vi "Lab Panel V6.00.vi"() -> ()   [LabVIEW 2017] (continued)
          n186 = local write "DISP LAB04-2"(w150) -> ()
        }
        frame #9 {
          w214 = 0
          w211 = FALSE
          # "initialise analog error control"
          n187 = local write "Resets Done"(0) -> ()
          n188 = local write "Auto Reset"(TRUE) -> ()
          n189 = local write "Er USB#0"(w214) -> ()
          n190 = local write "Er USB#1"(w214) -> ()
          n191 = local write "Er USB#2"(w214) -> ()
          n192 = local write "Analog error"(w211) -> ()
          n193 = local write "Reset Measuring"(w211) -> ()
          n194 = local write "Error USB #0"(w211) -> ()
          n195 = local write "Reset Error"(w211) -> ()
          n196 = local write "Error USB #1"(w211) -> ()
          n197 = local write "Error USB #2"(w211) -> ()
          n198 = local write "stop"(w211) -> ()
          n199 = local write "stop all"(w211) -> ()
        }
        frame #10 {
          # "get initial temperature values"
          n200 = stacked-sequence {
            frame #0 {
              w223 = T13 {"T1 Live"=20.0, "T1 Neut"=20.0, "T2 Live"=20.0, "T2 Neut"=20.0, "ID"=6.0, "ER"=10.0} ("LAB01 TEMP")
              n201 = local read "Select COM port"() -> (w218:refnum<visa-resource-name>)
              n202 = local write "LAB deg C"(w223) -> ()
              n203 = global write "Global display 4.vi" "LAB deg C"(w223) -> ()
              n204 = local write "OFF amps"(1.5) -> ()
              n205 = local write "ON amps"(20.0) -> ()
              n206 = local write "VOLTS"(250.0) -> ()
              n207 = local write "PF"(0.5) -> ()
              n208 = call "sub vi-open serial port v1.vi"("Select COM port"=w218) -> ("Error"=→"Com Port Status":bool, "LOOPS"=→"Com setup loops":i32, "VISA Com out"=→"VISA Com out":refnum<visa-resource-name>)  [unwired: 12 in]
            }
            frame #1 {
              n209 = for {
                N: 1 -> [_]
                w269 = TRUE
                n210 = local read "Temp Simulate"() -> (w225:bool)
                n211 = local write "Temp read loop"(0) -> ()
                n212 = case shown="True" w225 {
                  frame False {
                  }
                  frame True {
                    w271 = 20
                    n213 = local write "Ambient Volts"(2.92) -> ()
                    n214 = global write "Global display 3.vi" "Ref deg C"(w271) -> ()
                    n215 = local write "Ref deg C"(w271) -> ()
                  }
                }
                n216 = call "sub vi - GET ALL TEMP v7.vi"("LA01-EN"=w269, "LA02-EN"=w269, "LA03-EN"=w269, "LA04-EN"=w269, "LA05-EN"=w269, "simulate"=w225, "Gen Cal Value"=1) -> ("ID"=w231:T27, "LA01 TEMP"=w267:T28, "LA02 TEMP"=w260:T28, "LA04 TEMP"=w246:T28, "LA03 TEMP"=w253:T28, "LA05 TEMP"=w239:T28)  [unwired: 3 in, 4 out]
                n217 = local write "LAB05 TEMP"(w239) -> ()
                n218 = local write "LAB04 TEMP"(w246) -> ()
                n219 = Unbundle(w253) -> ("T1"=w250:dbl, "T2"=w249:dbl, "T3"=w248:dbl, "T4"=w247:dbl)  [unwired: 2 out]
                n220 = Unbundle(w267) -> ("T1"=w265:dbl, "T2"=w264:dbl, "T3"=w263:dbl, "T4"=w262:dbl)  [unwired: 2 out]
                n221 = Unbundle(w260) -> ("T1"=w257:dbl, "T2"=w256:dbl, "T3"=w255:dbl, "T4"=w254:dbl)  [unwired: 2 out]
                n222 = Unbundle(w246) -> ("T1"=w244:dbl, "T2"=w243:dbl, "T3"=w242:dbl, "T4"=w241:dbl)  [unwired: 2 out]
                n223 = Unbundle(w239) -> ("T1"=w237:dbl, "T2"=w236:dbl, "T3"=w235:dbl, "T4"=w234:dbl)  [unwired: 2 out]
                n224 = local write "LAB01 TEMP"(w267) -> ()
                n225 = local write "LAB02 TEMP"(w260) -> ()
                n226 = local write "LAB03 TEMP"(w253) -> ()
                n227 = Unbundle(w231) -> ("id1"=→"LAB01-TP":bool, "id2"=→"LAB02-TP":bool, "id3"=→"LAB03-TP":bool, "id4"=→"LAB04-TP":bool, "id5"=→"LAB05-TP":bool)
                n228 = local read "TEMP LA05"() -> (w238:T10)
                n229 = local read "TEMP LA04"() -> (w245:T10)
                n230 = local read "TEMP LA02"() -> (w259:T10)
                n231 = local read "TEMP LA03"() -> (w252:T10)
                n232 = local read "TEMP LA01"() -> (w266:T10)
                n233 = Bundle(cluster=w252, "TL-1"=w250, "TN-1"=w249, "TL-2"=w248, "TN-2"=w247) -> (w251:T10)  [unwired: 4 in]
                n234 = Bundle(cluster=w266, "TL-1"=w265, "TN-1"=w264, "TL-2"=w263, "TN-2"=w262) -> (w261:T10)  [unwired: 4 in]
                n235 = Bundle(cluster=w259, "TL-1"=w257, "TN-1"=w256, "TL-2"=w255, "TN-2"=w254) -> (w258:T10)  [unwired: 4 in]
                n236 = Bundle(cluster=w245, "TL-1"=w244, "TN-1"=w243, "TL-2"=w242, "TN-2"=w241) -> (w240:T10)  [unwired: 4 in]
                n237 = Bundle(cluster=w238, "TL-1"=w237, "TN-1"=w236, "TL-2"=w235, "TN-2"=w234) -> (w233:T10)  [unwired: 4 in]
                n238 = local write "TEMP LA03"(w251) -> ()
                n239 = local write "TEMP LA01"(w261) -> ()
                n240 = local write "TEMP LA02"(w258) -> ()
                n241 = local write "TEMP LA05"(w233) -> ()
                n242 = local write "TEMP LA04"(w240) -> ()
              }
            }
            frame #2 {
              w280 = 0
              n243 = local read "LAB01 TEMP"() -> (w282:T13)
              n244 = local read "SIG LAB01-2"() -> (w277:T2)
              n245 = Unbundle By Name(w282) -> ("T1 Live"=w275:dbl, "T1 Neut"=w274:dbl, "T2 Live"=w273:dbl, "T2 Neut"=w272:dbl)  [unwired: 2 out]
              n246 = local read "SIG LAB01-1"() -> (w279:T2)
              n247 = local read "TEMP LA01"() -> (w283:T10)
              n248 = Bundle By Name(cluster=w283, "TL-1"=w275, "TN-1"=w274, "TL-2"=w273, "TN-2"=w272, "TL -1COUNT"=w280, "TN-1 COUNT"=w280, "TL-2 COUNT"=w280, "TN-2 COUNT"=w280) -> (w281:T10)
              n249 = Bundle(cluster=w279, "Tmp Live"=w275, "Tmp Neut"=w274) -> (w278:T2)  [unwired: 3 in]
              n250 = Bundle(cluster=w277, "Tmp Live"=w273, "Tmp Neut"=w272) -> (w276:T2)  [unwired: 3 in]
              n251 = local write "SIG LAB01-2"(w276) -> ()
              n252 = local write "SIG LAB01-1"(w278) -> ()
              n253 = local write "TEMP LA01"(w281) -> ()
            }
            frame #3 {
              w292 = 0
              n254 = local read "LAB02 TEMP"() -> (w294:T13)
              n255 = Unbundle By Name(w294) -> ("T1 Live"=w287:dbl, "T1 Neut"=w286:dbl, "T2 Live"=w285:dbl, "T2 Neut"=w284:dbl)  [unwired: 2 out]
              n256 = local read "SIG LAB02-1"() -> (w291:T2)
              n257 = local read "SIG LAB02-2"() -> (w290:T2)
              n258 = local read "TEMP LA02"() -> (w295:T10)
              n259 = Bundle By Name(cluster=w295, "TL-1"=w287, "TN-1"=w286, "TL-2"=w285, "TN-2"=w284, "TL -1COUNT"=w292, "TN-1 COUNT"=w292, "TL-2 COUNT"=w292, "TN-2 COUNT"=w292) -> (w293:T10)
              n260 = Bundle(cluster=w290, "Tmp Live"=w285, "Tmp Neut"=w284) -> (w288:T2)  [unwired: 3 in]
              n261 = Bundle(cluster=w291, "Tmp Live"=w287, "Tmp Neut"=w286) -> (w289:T2)  [unwired: 3 in]
              n262 = local write "TEMP LA02"(w293) -> ()
              n263 = local write "SIG LAB02-1"(w289) -> ()
              n264 = local write "SIG LAB02-2"(w288) -> ()
            }
            frame #4 {
              w304 = 0
              n265 = local read "LAB03 TEMP"() -> (w306:T13)
              n266 = Unbundle By Name(w306) -> ("T1 Live"=w299:dbl, "T1 Neut"=w298:dbl, "T2 Live"=w297:dbl, "T2 Neut"=w296:dbl)  [unwired: 2 out]
              n267 = local read "SIG LAB03-1"() -> (w303:T2)
              n268 = local read "SIG LAB03-2"() -> (w302:T2)
              n269 = local read "TEMP LA03"() -> (w307:T10)
              n270 = Bundle By Name(cluster=w307, "TL-1"=w299, "TN-1"=w298, "TL-2"=w297, "TN-2"=w296, "TL -1COUNT"=w304, "TN-1 COUNT"=w304, "TL-2 COUNT"=w304, "TN-2 COUNT"=w304) -> (w305:T10)
              n271 = Bundle(cluster=w302, "Tmp Live"=w297, "Tmp Neut"=w296) -> (w300:T2)  [unwired: 3 in]
              n272 = Bundle(cluster=w303, "Tmp Live"=w299, "Tmp Neut"=w298) -> (w301:T2)  [unwired: 3 in]
              n273 = local write "TEMP LA03"(w305) -> ()
              n274 = local write "SIG LAB03-2"(w300) -> ()
              n275 = local write "SIG LAB03-1"(w301) -> ()
            }
            frame #5 {
              w316 = 0
              n276 = local read "LAB04 TEMP"() -> (w318:T13)
              n277 = Unbundle By Name(w318) -> ("T1 Live"=w311:dbl, "T1 Neut"=w310:dbl, "T2 Live"=w309:dbl, "T2 Neut"=w308:dbl)  [unwired: 2 out]
              n278 = local read "SIG LAB04-2"() -> (w314:T2)
              n279 = local read "SIG LAB04-1"() -> (w315:T2)
              n280 = local read "TEMP LA04"() -> (w319:T10)
              n281 = Bundle By Name(cluster=w319, "TL-1"=w311, "TN-1"=w310, "TL-2"=w309, "TN-2"=w308, "TL -1COUNT"=w316, "TN-1 COUNT"=w316, "TL-2 COUNT"=w316, "TN-2 COUNT"=w316) -> (w317:T10)
              n282 = Bundle(cluster=w314, "Tmp Live"=w309, "Tmp Neut"=w308) -> (w312:T2)  [unwired: 3 in]
              n283 = Bundle(cluster=w315, "Tmp Live"=w311, "Tmp Neut"=w310) -> (w313:T2)  [unwired: 3 in]
              n284 = local write "SIG LAB04-2"(w312) -> ()
              n285 = local write "TEMP LA04"(w317) -> ()
              n286 = local write "SIG LAB04-1"(w313) -> ()
            }
            frame #6 {
              w328 = 0
              n287 = local read "LAB05 TEMP"() -> (w330:T13)
              n288 = Unbundle By Name(w330) -> ("T1 Live"=w323:dbl, "T1 Neut"=w322:dbl, "T2 Live"=w321:dbl, "T2 Neut"=w320:dbl)  [unwired: 2 out]
              n289 = local read "SIG LAB05-2"() -> (w326:T2)
              n290 = local read "SIG LAB05-1"() -> (w327:T2)
              n291 = local read "TEMP LA05"() -> (w331:T10)
              n292 = Bundle By Name(cluster=w331, "TL-1"=w323, "TN-1"=w322, "TL-2"=w321, "TN-2"=w320, "TL -1COUNT"=w328, "TN-1 COUNT"=w328, "TL-2 COUNT"=w328, "TN-2 COUNT"=w328) -> (w329:T10)
              n293 = Bundle(cluster=w326, "Tmp Live"=w321, "Tmp Neut"=w320) -> (w324:T2)  [unwired: 3 in]
              n294 = Bundle(cluster=w327, "Tmp Live"=w323, "Tmp Neut"=w322) -> (w325:T2)  [unwired: 3 in]
              n295 = local write "SIG LAB05-2"(w324) -> ()
              n296 = local write "SIG LAB05-1"(w325) -> ()
              n297 = local write "TEMP LA05"(w329) -> ()
            }
          }
        }
        frame #11 {
          # "Create analog task"
          n298 = local read "DAQ Simulate"() -> (w333:bool)
          n299 = case shown="False" w333 {
            tunnel: w332 -> [w334 _]
            frame False {
              n300 = local read "RATE (Hz)"() -> (w341:dbl)
              n301 = local read "SAMPLES"() -> (w340:dbl)
              n302 = call "sub vi - AI USB4704 (3)  Create Task v4.vi"("Test"=w334, "Rate Hz"=w341, "Samples"=w340) -> ("physical channels 0"=→"physical channels 0":string, "physical channels 1"=→"physical channels 1":string, "physical channels 2"=→"physical channels 2":string, "TASK USB 0"=→"AI Task0":i32, "TASK USB 1"=→"AI Task1":i32, "TASK USB 2"=→"AI Task2":i32, "AI Task Er"=w338:bool)  [unwired: 5 in, 1 out]
              n303 = local write "Reset Error"(w338) -> ()
              "AI Task" <- TRUE
            }
            frame True {
            }
          }
        }
        frame #12 {
          # "Enable front panel, all settings done"
          n304 = property on="Tab Control 2" class="TabCtl (strict)"("DisabledEnum"=T17."Enabled" ("Disabled")) -> ()  [unwired: 2 in, 2 out]
          n305 = property on="Tab Control 2" class="TabCtl (strict)"("Value"=0) -> ()  [unwired: 2 in, 2 out]
        }
        frame #13 {
          n306 = property on="Tab Control 2" class="TabCtl (strict)"("Value"=0) -> ()  [unwired: 2 in, 2 out]
        }
      }
    }
    frame #2 {
      w349 = 250.0
      # "frames that only action on certain cycles, 13, 14, 15, 16, 19, 21"
      # "Main Loop"
      n307 = node-c288(w349) -> (w351:T19)  [unwired: 3 in]
      n308 = timed-loop {
        timing: w351 -> [_]
        timing-out: [_] -> w350
        tunnel: w349 -> [w353]
        tunnel: w348 -> [w352]
        i -> [w379]
        stop <- w354 stop-if-true
        n309 = node-c288() -> ()  [unwired: 1 in, 1 out]
        n310 = local read "Resets Done"() -> (w358:dbl)
        n311 = local read "SELECT LAB05-2"() -> (w359:T3)
        n312 = local read "SELECT LAB05-1"() -> (w360:T3)
        n313 = local read "SELECT LAB04-2"() -> (w361:T3)
        n314 = local read "SELECT LAB03-1"() -> (w364:T3)
        n315 = local read "SELECT LAB02-2"() -> (w365:T3)
        n316 = local read "SELECT LAB03-2"() -> (w363:T3)
        n317 = local read "SELECT LAB04-1"() -> (w362:T3)
        n318 = local read "SELECT LAB02-1"() -> (w366:T3)
        n319 = local read "run lab03-2"() -> (w373:bool)
        n320 = local read "run lab04-1"() -> (w372:bool)
        n321 = local read "run lab05-1"() -> (w370:bool)
        n322 = local read "run lab04-2"() -> (w371:bool)
        n323 = local read "run lab05-2"() -> (w369:bool)
        n324 = local read "run lab03-1"() -> (w374:bool)
        n325 = local read "run lab02-2"() -> (w375:bool)
        n326 = local read "SELECT LAB01-1"() -> (w368:T3)
        n327 = local read "SELECT LAB01-2"() -> (w367:T3)
        n328 = local read "run lab02-1"() -> (w376:bool)
        n329 = Greater?(x=w358, y=50) -> (0:w355:bool)
        n330 = Or(x=w355, y="stop") -> (x .or. y?=w354:bool)
        n331 = local read "run lab01-1"() -> (w378:bool)
        n332 = local read "run lab01-2"() -> (w377:bool)
        n333 = global write "Global display 1.vi" "stop disp"(w354) -> ()
        n334 = stacked-sequence {
          seq-local: [_ _ w496 _ _ _ _ _ _ _ _ _ _ _ _ _ _ _ _ _ _ _ _ _ _ _ _] -> [_ _ _ _ _ _ w2602 _ _ _ _ _ _ _ _ _ _ _ _ _ _ _ _ _ _ _ _]
          seq-local: [_ _ w495 _ _ _ _ _ _ _ _ _ _ _ _ _ _ _ _ _ _ _ _ _ _ _ _] -> [_ _ _ _ _ _ w2601 _ _ _ _ _ _ _ _ _ _ _ _ _ _ _ _ _ _ _ _]
          seq-local: [_ _ w482 _ _ _ _ _ _ _ _ _ _ _ _ _ _ _ _ _ _ _ _ _ _ _ _] -> [_ _ _ _ _ _ w2600 _ _ _ _ _ _ _ _ _ _ _ _ _ _ _ _ _ _ _ _]
          seq-local: [_ _ w481 _ _ _ _ _ _ _ _ _ _ _ _ _ _ _ _ _ _ _ _ _ _ _ _] -> [_ _ _ _ _ _ w2599 _ _ _ _ _ _ _ _ _ _ _ _ _ _ _ _ _ _ _ _]
          seq-local: [_ _ w480 _ _ _ _ _ _ _ _ _ _ _ _ _ _ _ _ _ _ _ _ _ _ _ _] -> [_ _ _ _ _ _ w2598 _ _ _ _ _ _ _ _ _ _ _ _ _ _ _ _ _ _ _ _]
          seq-local: [_ _ w479 _ _ _ _ _ _ _ _ _ _ _ _ _ _ _ _ _ _ _ _ _ _ _ _] -> [_ _ _ _ _ _ w2597 _ _ _ _ _ _ _ _ _ _ _ _ _ _ _ _ _ _ _ _]
          seq-local: [_ _ w478 _ _ _ _ _ _ _ _ _ _ _ _ _ _ _ _ _ _ _ _ _ _ _ _] -> [_ _ _ _ _ _ w2596 _ _ _ _ _ _ _ _ _ _ _ _ _ _ _ _ _ _ _ _]
          seq-local: [_ _ w477 _ _ _ _ _ _ _ _ _ _ _ _ _ _ _ _ _ _ _ _ _ _ _ _] -> [_ _ _ _ _ _ w2595 _ _ _ _ _ _ _ _ _ _ _ _ _ _ _ _ _ _ _ _]
          seq-local: [_ _ w476 _ _ _ _ _ _ _ _ _ _ _ _ _ _ _ _ _ _ _ _ _ _ _ _] -> [_ _ _ _ _ _ w2594 _ _ _ _ _ _ _ _ _ _ _ _ _ _ _ _ _ _ _ _]
          seq-local: [_ _ w475 _ _ _ _ _ _ _ _ _ _ _ _ _ _ _ _ _ _ _ _ _ _ _ _] -> [_ _ _ _ _ _ w2593 _ _ _ _ _ _ _ _ _ _ _ _ _ _ _ _ _ _ _ _]
          seq-local: [_ _ _ _ _ _ _ _ _ _ _ _ w3746 _ _ _ _ _ _ _ _ _ _ _ _ _ _] -> [_ _ _ _ _ _ _ _ _ _ _ _ _ w3783 _ _ _ _ _ _ _ _ _ _ _ _ _]
          seq-local: [w383 _ _ _ _ _ _ _ _ _ _ _ _ _ _ _ _ _ _ _ _ _ _ _ _ _ _] -> [_ _ _ _ _ _ _ _ _ _ _ _ _ _ _ _ _ _ _ _ _ _ _ _ _ _ w6492]
          tunnel: w378 -> [_ _ _ w513 w765 w2192 w2622 w2938 w3426 _ _ _ _ _ w4097 _ w5055 _ _ w5404 w5708 w5889 _ _ _ _ _]
          tunnel: w377 -> [_ _ _ w512 w763 w2191 w2621 w2939 w3425 _ _ _ _ _ w4096 _ w5053 _ _ w5403 w5707 w5887 _ _ _ _ _]
          tunnel: w376 -> [_ _ _ w511 w761 w2190 w2620 w2937 w3424 _ _ _ _ _ w4095 _ w5051 _ _ w5402 w5706 w5886 _ _ _ _ _]
          tunnel: w375 -> [_ _ _ w510 w759 w2189 w2619 w2936 w3423 _ _ _ _ _ w4094 _ w5049 _ _ w5401 w5705 w5885 _ _ _ _ _]
          tunnel: w374 -> [_ _ _ w509 w757 w2188 w2618 w2935 w3422 _ _ _ _ _ w4093 _ w5047 _ _ w5400 w5704 w5884 _ _ _ _ _]
          tunnel: w373 -> [_ _ _ w508 w755 w2187 w2617 w2934 w3421 _ _ _ _ _ w4092 _ w5045 _ _ w5399 w5703 w5883 _ _ _ _ _]
          tunnel: w372 -> [_ _ _ w507 w753 w2186 w2616 w2933 w3420 _ _ _ _ _ w4091 _ w5043 _ _ w5398 w5702 w5882 _ _ _ _ _]
          tunnel: w371 -> [_ _ _ w506 w751 w2185 w2615 w2932 w3419 _ _ _ _ _ w4090 _ w5041 _ _ w5397 w5701 w5881 _ _ _ _ _]
          tunnel: w370 -> [_ _ _ w505 w749 w2184 w2614 w2931 w3418 _ _ _ _ _ w4089 _ w5039 _ _ w5396 w5700 w5880 _ _ _ _ _]
          tunnel: w369 -> [_ _ _ w504 w747 w2183 w2613 w2930 w3417 _ _ _ _ _ w4088 _ w5037 _ _ w5395 w5699 w5879 _ _ _ _ _]
          tunnel: w368 -> [_ _ _ _ w764 w2182 w2612 _ _ _ _ _ _ _ _ _ w5057 _ _ _ _ _ w6352 _ _ _ _]
          tunnel: w367 -> [_ _ _ _ w762 w2181 w2611 _ _ _ _ _ _ _ _ _ w5052 _ _ _ _ _ w6351 _ _ _ _]
          tunnel: w366 -> [_ _ _ _ w760 w2180 w2610 _ _ _ _ _ _ _ _ _ w5050 _ _ _ _ _ w6350 _ _ _ _]
          tunnel: w365 -> [_ _ _ _ w758 w2179 w2609 _ _ _ _ _ _ _ _ _ w5048 _ _ _ _ _ w6349 _ _ _ _]
          tunnel: w364 -> [_ _ _ _ w756 w2178 w2608 _ _ _ _ _ _ _ _ _ w5046 _ _ _ _ _ w6348 _ _ _ _]
          tunnel: w363 -> [_ _ _ _ w754 w2177 w2607 _ _ _ _ _ _ _ _ _ w5044 _ _ _ _ _ w6347 _ _ _ _]
          tunnel: w362 -> [_ _ _ _ w752 w2176 w2606 _ _ _ _ _ _ _ _ _ w5042 _ _ _ _ _ w6346 _ _ _ _]
          tunnel: w361 -> [_ _ _ _ w750 w2175 w2605 _ _ _ _ _ _ _ _ _ w5040 _ _ _ _ _ w6345 _ _ _ _]
          tunnel: w360 -> [_ _ _ _ w748 w2174 w2604 _ _ _ _ _ _ _ _ _ w5038 _ _ _ _ _ w6344 _ _ _ _]
          tunnel: w359 -> [_ _ _ _ w746 w2173 w2603 _ _ _ _ _ _ _ _ _ w5036 _ _ _ _ _ w6343 _ _ _ _]
          tunnel: w355 -> [_ _ _ _ _ _ _ _ _ _ _ _ _ _ _ _ _ _ _ _ _ _ _ _ w6455 _ _]
          tunnel: w354 -> [_ _ _ _ _ _ _ _ _ _ _ _ _ _ _ _ _ _ _ _ _ _ _ _ w6454 _ _]
          tunnel: w353 -> [_ w428 _ _ _ _ _ _ _ _ _ _ _ _ _ _ _ _ _ _ _ _ _ _ _ _ _]
          tunnel: w352 -> [w382 _ _ w499 _ _ _ _ _ _ _ w3591 w3744 _ _ _ _ _ _ _ _ _ _ _ _ _ _]
          frame #0 {
            # "Acquire analog Inputs"
            n335 = Tick Count (ms)() -> (millisecond timer value=w383:u32)
            n336 = global write "Global 1.vi" "RATE(Hz)"("RATE (Hz)") -> ()
            n337 = local read "AI Task"() -> (w385:bool)
            n338 = case shown="True" w385 {
              tunnel: "RATE (Hz)" -> [_ _]
              tunnel: w382 -> [_ w394]
              tunnel: w382 -> [_ w393]
              frame False {
              }
              frame True {
                n339 = Tick Count (ms)() -> (millisecond timer value=w398:u32)
                n340 = flat-sequence {
                  tunnel: w398 -> [w400]
                  tunnel: [w400] -> w397
                  tunnel: w394 -> [w399]
                  tunnel: w397 -> [w409]
                  tunnel: [w407] -> w395
                  tunnel: [w414] -> w396
                  tunnel: w395 -> [w414]
                  tunnel: w393 -> [w412]
                  tunnel: w396 -> [w425]
                  frame #0 {
                    n341 = disable-structure shown="Disabled" {
                      disable-tunnel: w399 -> [w401 _]
                      frame Disabled {
                        n342 = local read "RATE (Hz)"() -> (w406:dbl)
                        n343 = local read "SAMPLES"() -> (w405:dbl)
                        n344 = call "sub vi - AI USB4704 (3)  Create Task v4.vi"("Test"=w401, "Rate Hz"=w406, "Samples"=w405) -> ("TASK USB 0"=w403:i32, "TASK USB 1"=w404:i32, "TASK USB 2"=w402:i32)  [unwired: 5 in, 5 out]
                        n345 = local write "AI Task0"(w403) -> ()
                        n346 = local write "AI Task1"(w404) -> ()
                        n347 = local write "AI Task2"(w402) -> ()
                      }
                      frame Enabled {
                      }
                    }
                  }
                  frame #1 {
                    n348 = Tick Count (ms)() -> (millisecond timer value=w407:u32)
                    n349 = Subtract(x=w407, y=w409) -> (x-y=→"ACQ Init TIme":u32)
                  }
                  frame #2 {
                    n350 = local read "SAMPLES"() -> (w415:dbl)
                    n351 = local read "AI Task0"() -> (w423:u64)
                    n352 = local read "AI Task1"() -> (w422:u32)
                    n353 = local read "AI Task2"() -> (w421:u32)
                    n354 = local read "MAIL SETTINGS"() -> (w413:T8)
                    n355 = call "sub vi - AI USB4704 (3) v73.vi"("Task0"=w423, "Test"=w412, "Task1"=w422, "Task2"=w421, "SAMPLES"=w415, "MAIL SETTINGS"=w413) -> ("Fault"=w410:bool, "data 0"=→"AI data 0" →"AI Data 0":waveform(dbl)[], "data 1"=→"AI data 1" →"AI Data 1":waveform(dbl)[], "data 2"=→"AI data 2" →"AI Data 2":waveform(dbl)[], "loop time"=→"AI loop time":dbl, "Fault Counts"=→"Analog Fault Counts":i32[], "error array"=→"AI Error":errorcluster[])  [unwired: 3 in]
                    n356 = local write "Analog error"(w410) -> ()
                  }
                  frame #3 {
                    n357 = Tick Count (ms)() -> (millisecond timer value=w426:u32)
                    n358 = Tick Count (ms)() -> ()  [unwired: 1 out]
                    n359 = Subtract(x=w426, y=w425) -> (x-y=→"ACQ Time":u32)
                  }
                }
              }
            }
            n360 = disable-structure shown="Disabled" {
              frame Disabled {
                n361 = call <userlib>:"Periodic Trigger__ogtk.vi"("time (ms)"=u32 1000) -> ("Triggered"=w387:bool)  [unwired: 12 in, 2 out]
                n362 = case shown="True" w387 {
                  frame False {
                  }
                  frame True {
                    n363 = control-ref of="This VI"() -> (w392:refnum<vi>)
                    n364 = invoke class="VI" method="FP.Get Image"(reference=w392) -> ("image data"=w391:T29)  [unwired: 5 in, 5 out]
                    n365 = Build Path(base path="path to JPEG file", name or relative path="FP.jpg") -> (appended path=w388:path)
                    n366 = call <vilib>:"Write JPEG File.vi"("image data"=w391, "path to JPEG file"=w388) -> ()  [unwired: 8 in, 2 out]
                  }
                }
              }
              frame Enabled {
              }
            }
          }
          frame #1 {
            w435 = FALSE
            # "Loop time (s)"
            # "set up cycle control"
            n367 = local read "jig cycle"() -> (w439:dbl)
            n368 = local read "Amps Fail level"() -> (w433:dbl)
            n369 = Divide(x=w428, y=1000.0) -> (x/y=w427:dbl)
            n370 = local read "DAQ Simulate"() -> (w430:bool)
            n371 = Divide(x="JIG ON TIME (S)", y=w427) -> (x/y=→"on loops":dbl)
            n372 = Divide(x="JIG OFF TIME (S)", y=w427) -> (x/y=→"off loops":dbl)
            n373 = Increment(x=w439) -> (x+1=w438:dbl)
            n374 = local write "Simulate IND"(w430) -> ()
            n375 = global write "Global display 3.vi" "Amps Fail"(w433) -> ()
            n376 = local write "TEMP"(w435) -> ()
            n377 = local write "AI"(w435) -> ()
            n378 = local read "Network Directory"() -> (w432:path)
            n379 = local write "jig cycle"(w438) -> ()
            n380 = call "sub vi - check network dir v2.vi"("PATH"=w432) -> ("error"=w431:bool)  [unwired: 10 in]
            n381 = disable-structure shown="Enabled" {
              frame Enabled {
                n382 = property on="Tab Control 2" class="TabCtl (strict)"() -> ("Pages"=w443:refnum<vi>[])  [unwired: 2 in, 2 out]
                n383 = Index Array(array=w443, index=8) -> (element=w445:refnum<vi>)
                n384 = property class="Page"(reference=w445, "PageVis"=TRUE) -> ()  [unwired: 1 in, 2 out]
              }
              frame Disabled {
              }
            }
            n385 = global write "Global display 3.vi" "network drive"(w431) -> ()
            n386 = event shown="[1] \"ADMIN\": Value Change" {
              selector: _ -> [_ _]
              dyn-events: _ -> [_ _]
              timeout: 10 -> [_ _]
              event Timeout {
                n387 = event-data() -> ()  [unwired: 1 in, 3 out]
              }
              event "ADMIN": Value Change {
                n388 = event-data() -> ()  [unwired: 1 in, 6 out]
                n389 = stacked-sequence {
                  seq-local: [_ w447 _] -> [_ _ w448]
                  frame #0 {
                    n390 = global write "Global 1.vi" "password"("9949") -> ()
                  }
                  frame #1 {
                    n391 = call "sub vi - password 1.vi"() -> ("RESULT"=w447:bool)  [unwired: 11 in]
                  }
                  frame #2 {
                    w450 = FALSE
                    n392 = property on="Tab Control 2" class="TabCtl (strict)"() -> ("Pages"=w454:refnum<vi>[])  [unwired: 2 in, 2 out]
                    n393 = Select(t=TRUE, s=w448, f=w450) -> (s? t:f=w449:bool)
                    n394 = Index Array(array=w454, index=8) -> (element=w452:refnum<vi>)
                    n395 = property class="Page"(reference=w452, "PageVis"=w449) -> ()  [unwired: 1 in, 2 out]
                    n396 = local write "ADMIN"(w450) -> ()
                  }
                }
              }
            }
            n397 = local write "network error"(w431) -> ()
          }
          frame #2 {
            w492 = 60.0
            # "Test Cycles"
            # "seconds"
            # "convert temperature rise minutes to cycles"
            n398 = local read "SET LAB05-2"() -> (w456:T5)
            n399 = local read "SET LAB05-1"() -> (w458:T5)
            n400 = local read "SET LAB04-2"() -> (w460:T5)
            n401 = local read "SET LAB01-1"() -> (w474:T6)
            n402 = local read "SET LAB01-2"() -> (w472:T5)
            n403 = local read "SET LAB02-2"() -> (w468:T5)
            n404 = local read "SET LAB04-1"() -> (w462:T5)
            n405 = local read "SET LAB03-1"() -> (w466:T5)
            n406 = local read "SET LAB03-2"() -> (w464:T5)
            n407 = local read "SET LAB02-1"() -> (w470:T5)
            n408 = local read "JIG OFF TIME (S)"() -> (w497:dbl)
            n409 = local read "JIG ON TIME (S)"() -> (w498:dbl)
            n410 = Unbundle By Name(w474) -> ("T-RISE mins"=w473:dbl)
            n411 = Unbundle(w456) -> ("T-RISE mins"=w455:dbl)  [unwired: 4 out]
            n412 = Unbundle(w458) -> ("T-RISE mins"=w457:dbl)  [unwired: 4 out]
            n413 = Unbundle(w460) -> ("T-RISE mins"=w459:dbl)  [unwired: 4 out]
            n414 = Unbundle(w472) -> ("T-RISE mins"=w471:dbl)  [unwired: 4 out]
            n415 = Unbundle(w470) -> ("T-RISE mins"=w469:dbl)  [unwired: 4 out]
            n416 = Unbundle(w462) -> ("T-RISE mins"=w461:dbl)  [unwired: 4 out]
            n417 = Unbundle(w468) -> ("T-RISE mins"=w467:dbl)  [unwired: 4 out]
            n418 = Unbundle(w464) -> ("T-RISE mins"=w463:dbl)  [unwired: 4 out]
            n419 = Unbundle(w466) -> ("T-RISE mins"=w465:dbl)  [unwired: 4 out]
            n420 = Add(x=w498, y=w497) -> (x+y=w491:dbl)
            n421 = Multiply(x=w492, y=w463) -> (x*y=w487:dbl)
            n422 = Multiply(x=w492, y=w461) -> (x*y=w486:dbl)
            n423 = Multiply(x=w492, y=w459) -> (x*y=w485:dbl)
            n424 = Multiply(x=w492, y=w457) -> (x*y=w484:dbl)
            n425 = Multiply(x=w492, y=w455) -> (x*y=w483:dbl)
            n426 = Multiply(x=w492, y=w471) -> (x*y=w493:dbl)
            n427 = Multiply(x=w492, y=w465) -> (x*y=w488:dbl)
            n428 = Multiply(x=w492, y=w473) -> (x*y=w494:dbl)
            n429 = Multiply(x=w492, y=w469) -> (x*y=w490:dbl)
            n430 = Multiply(x=w492, y=w467) -> (x*y=w489:dbl)
            n431 = Divide(x=w484, y=w491) -> (x/y=w476:dbl)
            n432 = Divide(x=w485, y=w491) -> (x/y=w477:dbl)
            n433 = Divide(x=w486, y=w491) -> (x/y=w478:dbl)
            n434 = Divide(x=w483, y=w491) -> (x/y=w475:dbl)
            n435 = Divide(x=w488, y=w491) -> (x/y=w480:dbl)
            n436 = Divide(x=w494, y=w491) -> (x/y=w496:dbl)
            n437 = Divide(x=w493, y=w491) -> (x/y=w495:dbl)
            n438 = Divide(x=w490, y=w491) -> (x/y=w482:dbl)
            n439 = Divide(x=w489, y=w491) -> (x/y=w481:dbl)
            n440 = Divide(x=w487, y=w491) -> (x/y=w479:dbl)
          }
          frame #3 {
            # "control cycle loops"
            n441 = local read "JIG OFF TIME (S)"() -> (w502:dbl)
            n442 = local read "JIG ON TIME (S)"() -> (w501:dbl)
            n443 = local read "on loops"() -> (w517:dbl)
            n444 = local read "off loops"() -> (w516:dbl)
            n445 = local read "jig cycle"() -> (w515:dbl)
            n446 = Add(x=w502, y=w501) -> (x+y=w500:dbl)
            n447 = Add(x=w517, y=w516) -> (x+y=w503:dbl)
            n448 = Greater Or Equal?(x=w515, y=w503) -> (x >= y?=w514:bool)
            n449 = case shown="True" w514 {
              tunnel: w513 -> [_ w552]
              tunnel: w512 -> [_ w551]
              tunnel: w511 -> [_ w550]
              tunnel: w510 -> [_ w549]
              tunnel: w509 -> [_ w548]
              tunnel: w508 -> [_ w547]
              tunnel: w507 -> [_ w546]
              tunnel: w506 -> [_ w545]
              tunnel: w505 -> [_ w544]
              tunnel: w504 -> [_ w543]
              tunnel: w500 -> [_ w542]
              tunnel: w499 -> [_ w518]
              frame False {
              }
              frame True {
                # "increment cycle value and convert cycles to minutes for temp rise"
                n450 = stacked-sequence {
                  tunnel: w518 -> [_ w556]
                  frame #0 {
                    n451 = local read "Temp read loop"() -> (w555:dbl)
                    n452 = Increment(x=w555) -> (x+1=w554:dbl)
                    n453 = local write "Temp read loop"(w554) -> ()
                  }
                  frame #1 {
                    n454 = case shown="True" w556 {
                      tunnel: [20 2] -> w558
                      frame False {
                      }
                      frame True {
                      }
                    }
                    n455 = local read "Temp read loop"() -> (w557:dbl)
                    n456 = Greater?(x=w557, y=w558) -> (0:w559:bool)
                    n457 = case shown="True" w559 {
                      frame False {
                      }
                      frame True {
                        n458 = local write "Temp read loop"(1) -> ()
                      }
                    }
                  }
                }
                n459 = local read "JIG RELAY CYCLES"() -> (w541:T9)
                n460 = local read "Temp read loop"() -> (→"Temp Up":dbl)
                n461 = Unbundle By Name(w541) -> ("LAB01-1"=w539:dbl, "LAB01-2"=w537:dbl, "LAB02-1"=w535:dbl, "LAB02-2"=w533:dbl, "LAB03-1"=w531:dbl, "LAB03-2"=w529:dbl, "LAB04-1"=w527:dbl, "LAB04-2"=w525:dbl, "LAB05-1"=w523:dbl, "LAB05-2"=w521:dbl)
                n462 = stacked-sequence {
                  tunnel: w552 -> [w573 _ _ _ _ _ _ _ _ _]
                  tunnel: w551 -> [_ w590 _ _ _ _ _ _ _ _]
                  tunnel: w550 -> [_ _ w607 _ _ _ _ _ _ _]
                  tunnel: w549 -> [_ _ _ w624 _ _ _ _ _ _]
                  tunnel: w548 -> [_ _ _ _ w641 _ _ _ _ _]
                  tunnel: w547 -> [_ _ _ _ _ w658 _ _ _ _]
                  tunnel: w546 -> [_ _ _ _ _ _ w675 _ _ _]
                  tunnel: w545 -> [_ _ _ _ _ _ _ w692 _ _]
                  tunnel: w544 -> [_ _ _ _ _ _ _ _ w709 _]
                  tunnel: w543 -> [_ _ _ _ _ _ _ _ _ w726]
                  tunnel: w542 -> [w570 w587 w604 w621 w638 w655 w672 w689 w706 w723]
                  tunnel: w539 -> [w564 _ _ _ _ _ _ _ _ _]
                  tunnel: [w563 _ _ _ _ _ _ _ _ _] -> w538
                  tunnel: w537 -> [_ w581 _ _ _ _ _ _ _ _]
                  tunnel: [_ w580 _ _ _ _ _ _ _ _] -> w536
                  tunnel: w535 -> [_ _ w598 _ _ _ _ _ _ _]
                  tunnel: [_ _ w597 _ _ _ _ _ _ _] -> w534
                  tunnel: w533 -> [_ _ _ w615 _ _ _ _ _ _]
                  tunnel: [_ _ _ w614 _ _ _ _ _ _] -> w532
                  tunnel: w531 -> [_ _ _ _ w632 _ _ _ _ _]
                  tunnel: [_ _ _ _ w631 _ _ _ _ _] -> w530
                  tunnel: w529 -> [_ _ _ _ _ w649 _ _ _ _]
                  tunnel: [_ _ _ _ _ w648 _ _ _ _] -> w528
                  tunnel: w527 -> [_ _ _ _ _ _ w666 _ _ _]
                  tunnel: [_ _ _ _ _ _ w665 _ _ _] -> w526
                  tunnel: w525 -> [_ _ _ _ _ _ _ w683 _ _]
                  tunnel: [_ _ _ _ _ _ _ w682 _ _] -> w524
                  tunnel: w523 -> [_ _ _ _ _ _ _ _ w700 _]
                  tunnel: [_ _ _ _ _ _ _ _ w699 _] -> w522
                  tunnel: w521 -> [_ _ _ _ _ _ _ _ _ w717]
                  tunnel: [_ _ _ _ _ _ _ _ _ w716] -> w520
                  frame #0 {
                    n463 = local read "DISP LAB01-1"() -> (w568:T4)
                    n464 = Unbundle By Name(w568) -> ("CYCLE"=w569:dbl)
                    n465 = case shown="True" w573 {
                      tunnel: w569 -> [w575 w579]
                      tunnel: [w575 w578] -> w567
                      tunnel: w564 -> [w574 w577]
                      tunnel: [w574 w576] -> w563
                      frame False {
                      }
                      frame True {
                        n466 = Increment(x=w577) -> (x+1=w576:dbl)
                        n467 = Increment(x=w579) -> (x+1=w578:dbl)
                      }
                    }
                    n468 = Multiply(x=w567, y=w570) -> (x*y=w571:dbl)
                    n469 = Divide(x=w571, y=60.0) -> (x/y=w566:dbl)
                    n470 = Bundle By Name(cluster=w568, "CYCLE"=w567, "MINS"=w566) -> (w565:T4)
                    n471 = local write "DISP LAB01-1"(w565) -> ()
                  }
                  frame #1 {
                    n472 = local read "DISP LAB01-2"() -> (w585:T4)
                    n473 = Unbundle By Name(w585) -> ("CYCLE"=w586:dbl)
                    n474 = case shown="True" w590 {
                      tunnel: w586 -> [w592 w596]
                      tunnel: [w592 w595] -> w583
                      tunnel: w581 -> [w591 w594]
                      tunnel: [w591 w593] -> w580
                      frame False {
                      }
                      frame True {
                        n475 = Increment(x=w594) -> (x+1=w593:dbl)
                        n476 = Increment(x=w596) -> (x+1=w595:dbl)
                      }
                    }
                    n477 = Multiply(x=w583, y=w587) -> (x*y=w588:dbl)
                    n478 = Divide(x=w588, y=60.0) -> (x/y=w582:dbl)
                    n479 = Bundle By Name(cluster=w585, "CYCLE"=w583, "MINS"=w582) -> (w584:T4)
                    n480 = local write "DISP LAB01-2"(w584) -> ()
                  }
                  frame #2 {
                    n481 = local read "DISP LAB02-1"() -> (w602:T4)
                    n482 = Unbundle By Name(w602) -> ("CYCLE"=w603:dbl)
                    n483 = case shown="True" w607 {
                      tunnel: [w609 w613] -> w600
                      tunnel: w603 -> [w609 w612]
                      tunnel: w598 -> [w608 w611]
                      tunnel: [w608 w610] -> w597
                      frame False {
                      }
                      frame True {
                        n484 = Increment(x=w611) -> (x+1=w610:dbl)
                        n485 = Increment(x=w612) -> (x+1=w613:dbl)
                      }
                    }
                    n486 = Multiply(x=w600, y=w604) -> (x*y=w605:dbl)
                    n487 = Divide(x=w605, y=60.0) -> (x/y=w599:dbl)
                    n488 = Bundle By Name(cluster=w602, "CYCLE"=w600, "MINS"=w599) -> (w601:T4)
                    n489 = local write "DISP LAB02-1"(w601) -> ()
                  }
                  frame #3 {
                    n490 = local read "DISP LAB02-2"() -> (w619:T4)
                    n491 = Unbundle By Name(w619) -> ("CYCLE"=w620:dbl)
                    n492 = case shown="True" w624 {
                      tunnel: [w626 w630] -> w618
                      tunnel: w620 -> [w626 w629]
                      tunnel: w615 -> [w625 w628]
                      tunnel: [w625 w627] -> w614
                      frame False {
                      }
                      frame True {
                        n493 = Increment(x=w628) -> (x+1=w627:dbl)
                        n494 = Increment(x=w629) -> (x+1=w630:dbl)
                      }
                    }
                    n495 = Multiply(x=w618, y=w621) -> (x*y=w622:dbl)
                    n496 = Divide(x=w622, y=60.0) -> (x/y=w617:dbl)
                    n497 = Bundle By Name(cluster=w619, "CYCLE"=w618, "MINS"=w617) -> (w616:T4)
                    n498 = local write "DISP LAB02-2"(w616) -> ()
                  }
                  frame #4 {
                    n499 = local read "DISP LAB03-1"() -> (w636:T4)
                    n500 = Unbundle(w636) -> ("CYCLE"=w637:dbl)  [unwired: 2 out]
                    n501 = case shown="True" w641 {
                      tunnel: [w643 w647] -> w633
                      tunnel: w637 -> [w643 w646]
                      tunnel: w632 -> [w642 w645]
                      tunnel: [w642 w644] -> w631
                      frame False {
                      }
                      frame True {
                        n502 = Increment(x=w645) -> (x+1=w644:dbl)
                        n503 = Increment(x=w646) -> (x+1=w647:dbl)
                      }
                    }
                    n504 = Multiply(x=w633, y=w638) -> (x*y=w639:dbl)
                    n505 = Divide(x=w639, y=60.0) -> (x/y=w634:dbl)
                    n506 = Bundle(cluster=w636, "CYCLE"=w633, "MINS"=w634) -> (w635:T4)  [unwired: 1 in]
                    n507 = local write "DISP LAB03-1"(w635) -> ()
                  }
                  frame #5 {
                    n508 = local read "DISP LAB03-2"() -> (w653:T4)
                    n509 = Unbundle(w653) -> ("CYCLE"=w654:dbl)  [unwired: 2 out]
                    n510 = case shown="True" w658 {
                      tunnel: [w660 w664] -> w652
                      tunnel: w654 -> [w660 w663]
                      tunnel: w649 -> [w659 w662]
                      tunnel: [w659 w661] -> w648
                      frame False {
                      }
                      frame True {
                        n511 = Increment(x=w662) -> (x+1=w661:dbl)
                        n512 = Increment(x=w663) -> (x+1=w664:dbl)
                      }
                    }
                    n513 = Multiply(x=w652, y=w655) -> (x*y=w656:dbl)
                    n514 = Divide(x=w656, y=60.0) -> (x/y=w651:dbl)
                    n515 = Bundle(cluster=w653, "CYCLE"=w652, "MINS"=w651) -> (w650:T4)  [unwired: 1 in]
                    n516 = local write "DISP LAB03-2"(w650) -> ()
                  }
                  frame #6 {
                    n517 = local read "DISP LAB04-1"() -> (w670:T4)
                    n518 = Unbundle(w670) -> ("CYCLE"=w671:dbl)  [unwired: 2 out]
                    n519 = case shown="True" w675 {
                      tunnel: [w677 w681] -> w668
                      tunnel: w671 -> [w677 w680]
                      tunnel: w666 -> [w676 w679]
                      tunnel: [w676 w678] -> w665
                      frame False {
                      }
                      frame True {
                        n520 = Increment(x=w679) -> (x+1=w678:dbl)
                        n521 = Increment(x=w680) -> (x+1=w681:dbl)
                      }
                    }
                    n522 = Multiply(x=w668, y=w672) -> (x*y=w673:dbl)
                    n523 = Divide(x=w673, y=60.0) -> (x/y=w667:dbl)
                    n524 = Bundle(cluster=w670, "CYCLE"=w668, "MINS"=w667) -> (w669:T4)  [unwired: 1 in]
                    n525 = local write "DISP LAB04-1"(w669) -> ()
                  }
                  frame #7 {
                    n526 = local read "DISP LAB04-2"() -> (w687:T4)
                    n527 = Unbundle(w687) -> ("CYCLE"=w688:dbl)  [unwired: 2 out]
                    n528 = case shown="True" w692 {
                      tunnel: [w694 w698] -> w685
                      tunnel: w688 -> [w694 w697]
                      tunnel: w683 -> [w693 w696]
                      tunnel: [w693 w695] -> w682
                      frame False {
                      }
                      frame True {
                        n529 = Increment(x=w696) -> (x+1=w695:dbl)
                        n530 = Increment(x=w697) -> (x+1=w698:dbl)
                      }
                    }
                    n531 = Multiply(x=w685, y=w689) -> (x*y=w691:dbl)
                    n532 = Divide(x=w691, y=60.0) -> (x/y=w684:dbl)
                    n533 = Bundle(cluster=w687, "CYCLE"=w685, "MINS"=w684) -> (w686:T4)  [unwired: 1 in]
                    n534 = local write "DISP LAB04-2"(w686) -> ()
                  }
                  frame #8 {
                    n535 = local read "DISP LAB05-1"() -> (w704:T4)
                    n536 = Unbundle(w704) -> ("CYCLE"=w705:dbl)  [unwired: 2 out]
                    n537 = case shown="True" w709 {
                      tunnel: [w711 w715] -> w702
                      tunnel: w705 -> [w711 w714]
                      tunnel: w700 -> [w710 w713]
                      tunnel: [w710 w712] -> w699
                      frame False {
                      }
                      frame True {
                        n538 = Increment(x=w713) -> (x+1=w712:dbl)
                        n539 = Increment(x=w714) -> (x+1=w715:dbl)
                      }
                    }
                    n540 = Multiply(x=w702, y=w706) -> (x*y=w707:dbl)
                    n541 = Divide(x=w707, y=60.0) -> (x/y=w701:dbl)
                    n542 = Bundle(cluster=w704, "CYCLE"=w702, "MINS"=w701) -> (w703:T4)  [unwired: 1 in]
                    n543 = local write "DISP LAB05-1"(w703) -> ()
                  }
                  frame #9 {
                    n544 = local read "DISP LAB05-2"() -> (w722:T4)
                    n545 = Unbundle(w722) -> ("CYCLE"=w721:dbl)  [unwired: 2 out]
                    n546 = case shown="True" w726 {
                      tunnel: [w728 w732] -> w720
                      tunnel: w721 -> [w728 w731]
                      tunnel: w717 -> [w727 w730]
                      tunnel: [w727 w729] -> w716
                      frame False {
                      }
                      frame True {
                        n547 = Increment(x=w730) -> (x+1=w729:dbl)
                        n548 = Increment(x=w731) -> (x+1=w732:dbl)
                      }
                    }
                    n549 = Multiply(x=w720, y=w723) -> (x*y=w724:dbl)
                    n550 = Divide(x=w724, y=60.0) -> (x/y=w719:dbl)
                    n551 = Bundle(cluster=w722, "CYCLE"=w720, "MINS"=w719) -> (w718:T4)  [unwired: 1 in]
                    n552 = local write "DISP LAB05-2"(w718) -> ()
                  }
                }
                n553 = local write "jig cycle"(0) -> ()
                n554 = Bundle By Name(cluster=w541, "LAB01-1"=w538, "LAB01-2"=w536, "LAB02-1"=w534, "LAB02-2"=w532, "LAB03-1"=w530, "LAB03-2"=w528, "LAB04-1"=w526, "LAB04-2"=w524, "LAB05-1"=w522, "LAB05-2"=w520) -> (w540:T9)
                n555 = local write "JIG RELAY CYCLES"(w540) -> ()
              }
            }
          }
          frame #4 {
            # "Note : Run lab0X-N variables are set which are written to digital I/O in frame 11"
            # "Why are these here?"
            # "START & STOP test RUN switch change, start test if true and stop test if false"
            n556 = Get Date/Time In Seconds() -> (seconds since 1Jan1904=w744:timestamp)
            n557 = local read "C drive data root dir"() -> (w737:path)
            n558 = Format Date/Time String(time format string (%c)="%b\\%a%d", seconds (now)=w744) -> (date/time string=w768:string)  [unwired: 1 in]
            n559 = Format Date/Time String(time format string (%c)="%H%M", seconds (now)=w744) -> (date/time string=w766:string)  [unwired: 1 in]
            n560 = Format Date/Time String(time format string (%c)="LabPanel%Y", seconds (now)=w744) -> (date/time string=w743:string)  [unwired: 1 in]
            n561 = Path To String(path=w737) -> (string=w740:string)
            n562 = global write "Global 1.vi" "C drive root path"(w737) -> ()
            n563 = local read "Ref deg C"() -> (w733:dbl)
            n564 = Concatenate Strings(w740, "\\") -> (w738:string)
            n565 = event shown="[1] \"RUN LAB01-1\": Value Change" {
              selector: _ -> [_ _ _ _ _ _ _ _ _ _ _]
              dyn-events: _ -> [_ _ _ _ _ _ _ _ _ _ _]
              timeout: 10 -> [_ _ _ _ _ _ _ _ _ _ _]
              tunnel: w738 -> [_ w781 w921 w1062 w1202 w1342 w1482 w1622 w1762 w1902 w2043]
              tunnel: w768 -> [_ w780 w920 w1061 w1201 w1341 w1481 w1621 w1761 w1901 w2042]
              tunnel: w766 -> [_ w778 w919 w1060 w1200 w1340 w1480 w1620 w1760 w1900 w2041]
              tunnel: w764 -> [_ w779 _ _ _ _ _ _ _ _ _]
              tunnel: w765 -> [_ _ _ _ _ _ _ _ _ _ _]
              tunnel: w763 -> [_ _ _ _ _ _ _ _ _ _ _]
              tunnel: w762 -> [_ _ w918 _ _ _ _ _ _ _ _]
              tunnel: w761 -> [_ _ _ _ _ _ _ _ _ _ _]
              tunnel: w760 -> [_ _ _ w1059 _ _ _ _ _ _ _]
              tunnel: w759 -> [_ _ _ _ _ _ _ _ _ _ _]
              tunnel: w758 -> [_ _ _ _ w1199 _ _ _ _ _ _]
              tunnel: w757 -> [_ _ _ _ _ _ _ _ _ _ _]
              tunnel: w756 -> [_ _ _ _ _ w1339 _ _ _ _ _]
              tunnel: w755 -> [_ _ _ _ _ _ _ _ _ _ _]
              tunnel: w754 -> [_ _ _ _ _ _ w1479 _ _ _ _]
              tunnel: w753 -> [_ _ _ _ _ _ _ _ _ _ _]
              tunnel: w752 -> [_ _ _ _ _ _ _ w1619 _ _ _]
              tunnel: w751 -> [_ _ _ _ _ _ _ _ _ _ _]
              tunnel: w750 -> [_ _ _ _ _ _ _ _ w1759 _ _]
              tunnel: w749 -> [_ _ _ _ _ _ _ _ _ _ _]
              tunnel: w748 -> [_ _ _ _ _ _ _ _ _ w1899 _]
              tunnel: w747 -> [_ _ _ _ _ _ _ _ _ _ _]
              tunnel: w746 -> [_ _ _ _ _ _ _ _ _ _ w2040]
              tunnel: w743 -> [_ w777 w917 w1058 w1198 w1338 w1478 w1618 w1758 w1898 w2039]
              tunnel: [_ w776 w916 w1057 w1197 w1337 w1477 w1617 w1757 w1897 w2038] -> w741
              tunnel: "RESET CYCLES TO ZERO?" -> [_ w775 w914 w1055 w1195 w1335 w1475 w1615 w1755 w1895 w2036]
              tunnel: "YES" -> [_ w774 w913 w1054 w1194 w1334 w1474 w1614 w1754 w1894 w2035]
              tunnel: "NO" -> [_ w773 w912 w1053 w1193 w1333 w1473 w1613 w1753 w1893 w2034]
              tunnel: w733 -> [_ w770 w911 w1051 w1192 w1332 w1472 w1612 w1752 w1892 w2032]
              event Timeout {
                n566 = event-data() -> ()  [unwired: 1 in, 3 out]
              }
              event "RUN LAB01-1": Value Change {
                n567 = event-data() -> ("NewVal"=w771:bool)  [unwired: 1 in, 5 out]
                n568 = local read "SIG LAB01-1"() -> (w772:T2)
                n569 = local write "run lab01-1"(w771) -> ()
                n570 = case shown="True" w771 {
                  tunnel: w781 -> [_ w819]
                  tunnel: w780 -> [_ w818]
                  tunnel: w779 -> [w783 w817]
                  tunnel: w778 -> [_ w816]
                  tunnel: w777 -> [_ w815]
                  tunnel: [w782 w814] -> w776
                  tunnel: w775 -> [_ w813]
                  tunnel: w774 -> [_ w812]
                  tunnel: w773 -> [_ w811]
                  tunnel: w772 -> [_ w810]
                  tunnel: w770 -> [_ w809]
                  frame False {
                    # "stop test"
                    n571 = stacked-sequence {
                      tunnel: w783 -> [_ w795 _]
                      tunnel: [_ w787 _] -> w782
                      frame #0 {
                        n572 = local read "DISP LAB01-1"() -> (w786:T4)
                        n573 = Bundle(cluster=w786, "STATUS"="STOP") -> (w784:T4)  [unwired: 2 in]
                        n574 = local write "DISP LAB01-1"(w784) -> ()
                      }
                      frame #1 {
                        n575 = local read "DISP LAB01-1"() -> (w794:T4)
                        n576 = Unbundle(w794) -> ("CYCLE"=w792:dbl, "MINS"=w793:dbl)  [unwired: 1 out]
                        n577 = case shown="\"CYCLE TEST\"" w795 {
                          tunnel: w793 -> [_ _ w802]
                          tunnel: w792 -> [w800 w801 _]
                          tunnel: [w800 w801 w802] -> w791
                          frame "CHART TEST", Default {
                          }
                          frame "CYCLE TEST" {
                          }
                          frame "T-RISE TEST" {
                          }
                        }
                        n578 = local read "TDMS LAB01-1"() -> (w799:refnum<k34>)
                        n579 = Build Array("STOPPED") -> (w796:string[])
                        n580 = Build Array(w791) -> (w790:dbl[])
                        n581 = TDMS Write(0:w799, 5:"TEST RESULT", 7:w796, 9:w790) -> (4:w788:refnum<k34>, 15:w789:errorcluster)  [unwired: 2 in, 2 out]
                        n582 = TDMS Close(8:w789, 11:w788) -> (0:w787:errorcluster)  [unwired: 1 out]
                      }
                      frame #2 {
                        n583 = stacked-sequence {
                          tunnel: "LAB01-1" -> [w805 w807]
                          frame #0 {
                            n584 = call "sub vi - defrag tdms v1.vi"("panel id"=w805) -> ("error out"=w804:errorcluster)  [unwired: 10 in]
                            n585 = local write "data file error"(w804) -> ()
                          }
                          frame #1 {
                            n586 = call "Save data file (stop) v3.vi"("panel id"=w807) -> ("network file save error"=w806:errorcluster)  [unwired: 9 in, 1 out]
                            n587 = local write "RESULT LAB01-1"(FALSE) -> ()
                            n588 = local write "data file error"(w806) -> ()
                          }
                        }
                      }
                    }
                  }
                  frame True {
                    n589 = stacked-sequence {
                      seq-local: [w821 _] -> [_ w825]
                      tunnel: w819 -> [_ w835]
                      tunnel: w818 -> [_ w834]
                      tunnel: w817 -> [_ w833]
                      tunnel: w816 -> [_ w832]
                      tunnel: w815 -> [_ w831]
                      tunnel: [_ w830] -> w814
                      tunnel: w813 -> [_ w829]
                      tunnel: w812 -> [_ w828]
                      tunnel: w811 -> [_ w827]
                      tunnel: w810 -> [w823 w826]
                      tunnel: w809 -> [_ w824]
                      frame #0 {
                        n590 = Unbundle(w823) -> ("AMPS"=w822:dbl)  [unwired: 4 out]
                        n591 = call "Check For Amps on v1.vi"("ID"="LAB01-1", "amps"=w822) -> ("amps"=w821:bool)  [unwired: 9 in]
                      }
                      frame #1 {
                        n592 = case shown="True" w825 {
                          tunnel: w835 -> [_ w848]
                          tunnel: w834 -> [_ w847]
                          tunnel: w833 -> [_ w846]
                          tunnel: w832 -> [_ w845]
                          tunnel: w831 -> [_ w844]
                          tunnel: [errorcluster {"status"=FALSE, "code"=0, "source"=""} ("error out") w843] -> w830
                          tunnel: w829 -> [_ w842]
                          tunnel: w828 -> [_ w841]
                          tunnel: w827 -> [_ w840]
